vi "Frame_to_word_14444B.vi"() -> ()   [LabVIEW 2019]
uses:
  <vilib>/addons/Modulation/Analog/support/mod_Set Error Source.vi
  <vilib>/addons/Modulation/Digital/Support/Common/Validators/mod_Generate Filter Coefficients Validate.vi
  <vilib>/addons/Modulation/Digital/General/subVIs/mod_Generate Filter Coefficients.vi
  <vilib>/addons/Modulation/Digital/General/MT Generate ASK system parameters (M).vi
  <vilib>/addons/Modulation/Analog/MT Modulate AM (DSB).vi
  <vilib>/addons/Modulation/Analog/MT Upconvert Baseband (Real).vi
  <vilib>/measure/macond.llb/IIR Filter for 1 Chan.vi
  <vilib>/express/express analysis/Spectral/Block/exnSpectralBlock spectral measurements RMS poly.vi
  <vilib>/express/express analysis/Spectral/Block/exnSpectralBlock spectral measurements RMS WFM.vi
  <vilib>/addons/Modulation/Analog/MT Downconvert Passband (Real).vi
  <vilib>/addons/Modulation/Analog/MT Demodulate AM (DSB).vi
  <vilib>/ErrorRing/Error Ring.xnode
  <vilib>/express/express analysis/Spectral/XNode/ExpressSpectralMeasurementsBlockNode.xnode
  <vilib>/addons/Modulation/niAMT.lvlib
  <vilib>/measure/NI_MAPro.lvlib
  <vilib>/addons/Modulation/niDMT.lvlib
panel:
  out "lo(x)":u8 format="%x"
  out "hi(x)":u8 format="%x"
  out "Array of byte":u8[](array[numeric]) format="%x"
  out "decode":cluster{"t0":dbl, "dt":dbl, "Y":dbl[]}(graph)
  out "Command":cluster{"t0":dbl, "dt":dbl, "Y":dbl[]}(graph)
  out "DEMODulate":cluster{"t0":dbl, "dt":dbl, "Y":dbl[]}(graph)
  out "spectrum analog signal 6":waveform(dbl)(graph)
  out "spectrum analog signal 5":cluster{"t0":dbl, "dt":dbl, "Y":dbl[]}(graph)
  out "Analog signal 8":waveform(dbl)(graph)
  out "spectrum analog signal 4":cluster{"t0":dbl, "dt":dbl, "Y":dbl[]}(graph)
  out "antenna":waveform(dbl)(graph)
  out "summ":waveform(dbl)(graph)
  out "antenna":waveform(dbl)(graph)
  out "spectrum analog signal 3":cluster{"t0":dbl, "dt":dbl, "Y":dbl[]}(graph)
  out "spectrum analog signal 2":cluster{"t0":dbl, "dt":dbl, "Y":dbl[]}(graph)
  out "spectrum analog signal":cluster{"t0":dbl, "dt":dbl, "Y":dbl[]}(graph)
  out "Video  without CRC":cluster{"t0":dbl, "dt":dbl, "Y":dbl[]}(graph)
  in  "AFi":u8[](array[numeric])=[2] format="%x"
  in  "APf":u8[](array[numeric])=[5] format="%x"
  out "SOF+DATA+EOF":cluster{"t0":dbl, "dt":dbl, "Y":dbl[]}(graph)
  out "Video":cluster{"t0":dbl, "dt":dbl, "Y":dbl[]}(graph)
  out "video NRZ":cluster{"t0":dbl, "dt":dbl, "Y":dbl[]}(graph)
  in  "command":enum16{"WUPB", "REQB"}(ring)
  in  "CARRIER (hz)":dbl
  in  "BIT RATE":dbl
  out "10% ASK":waveform(dbl)(graph)
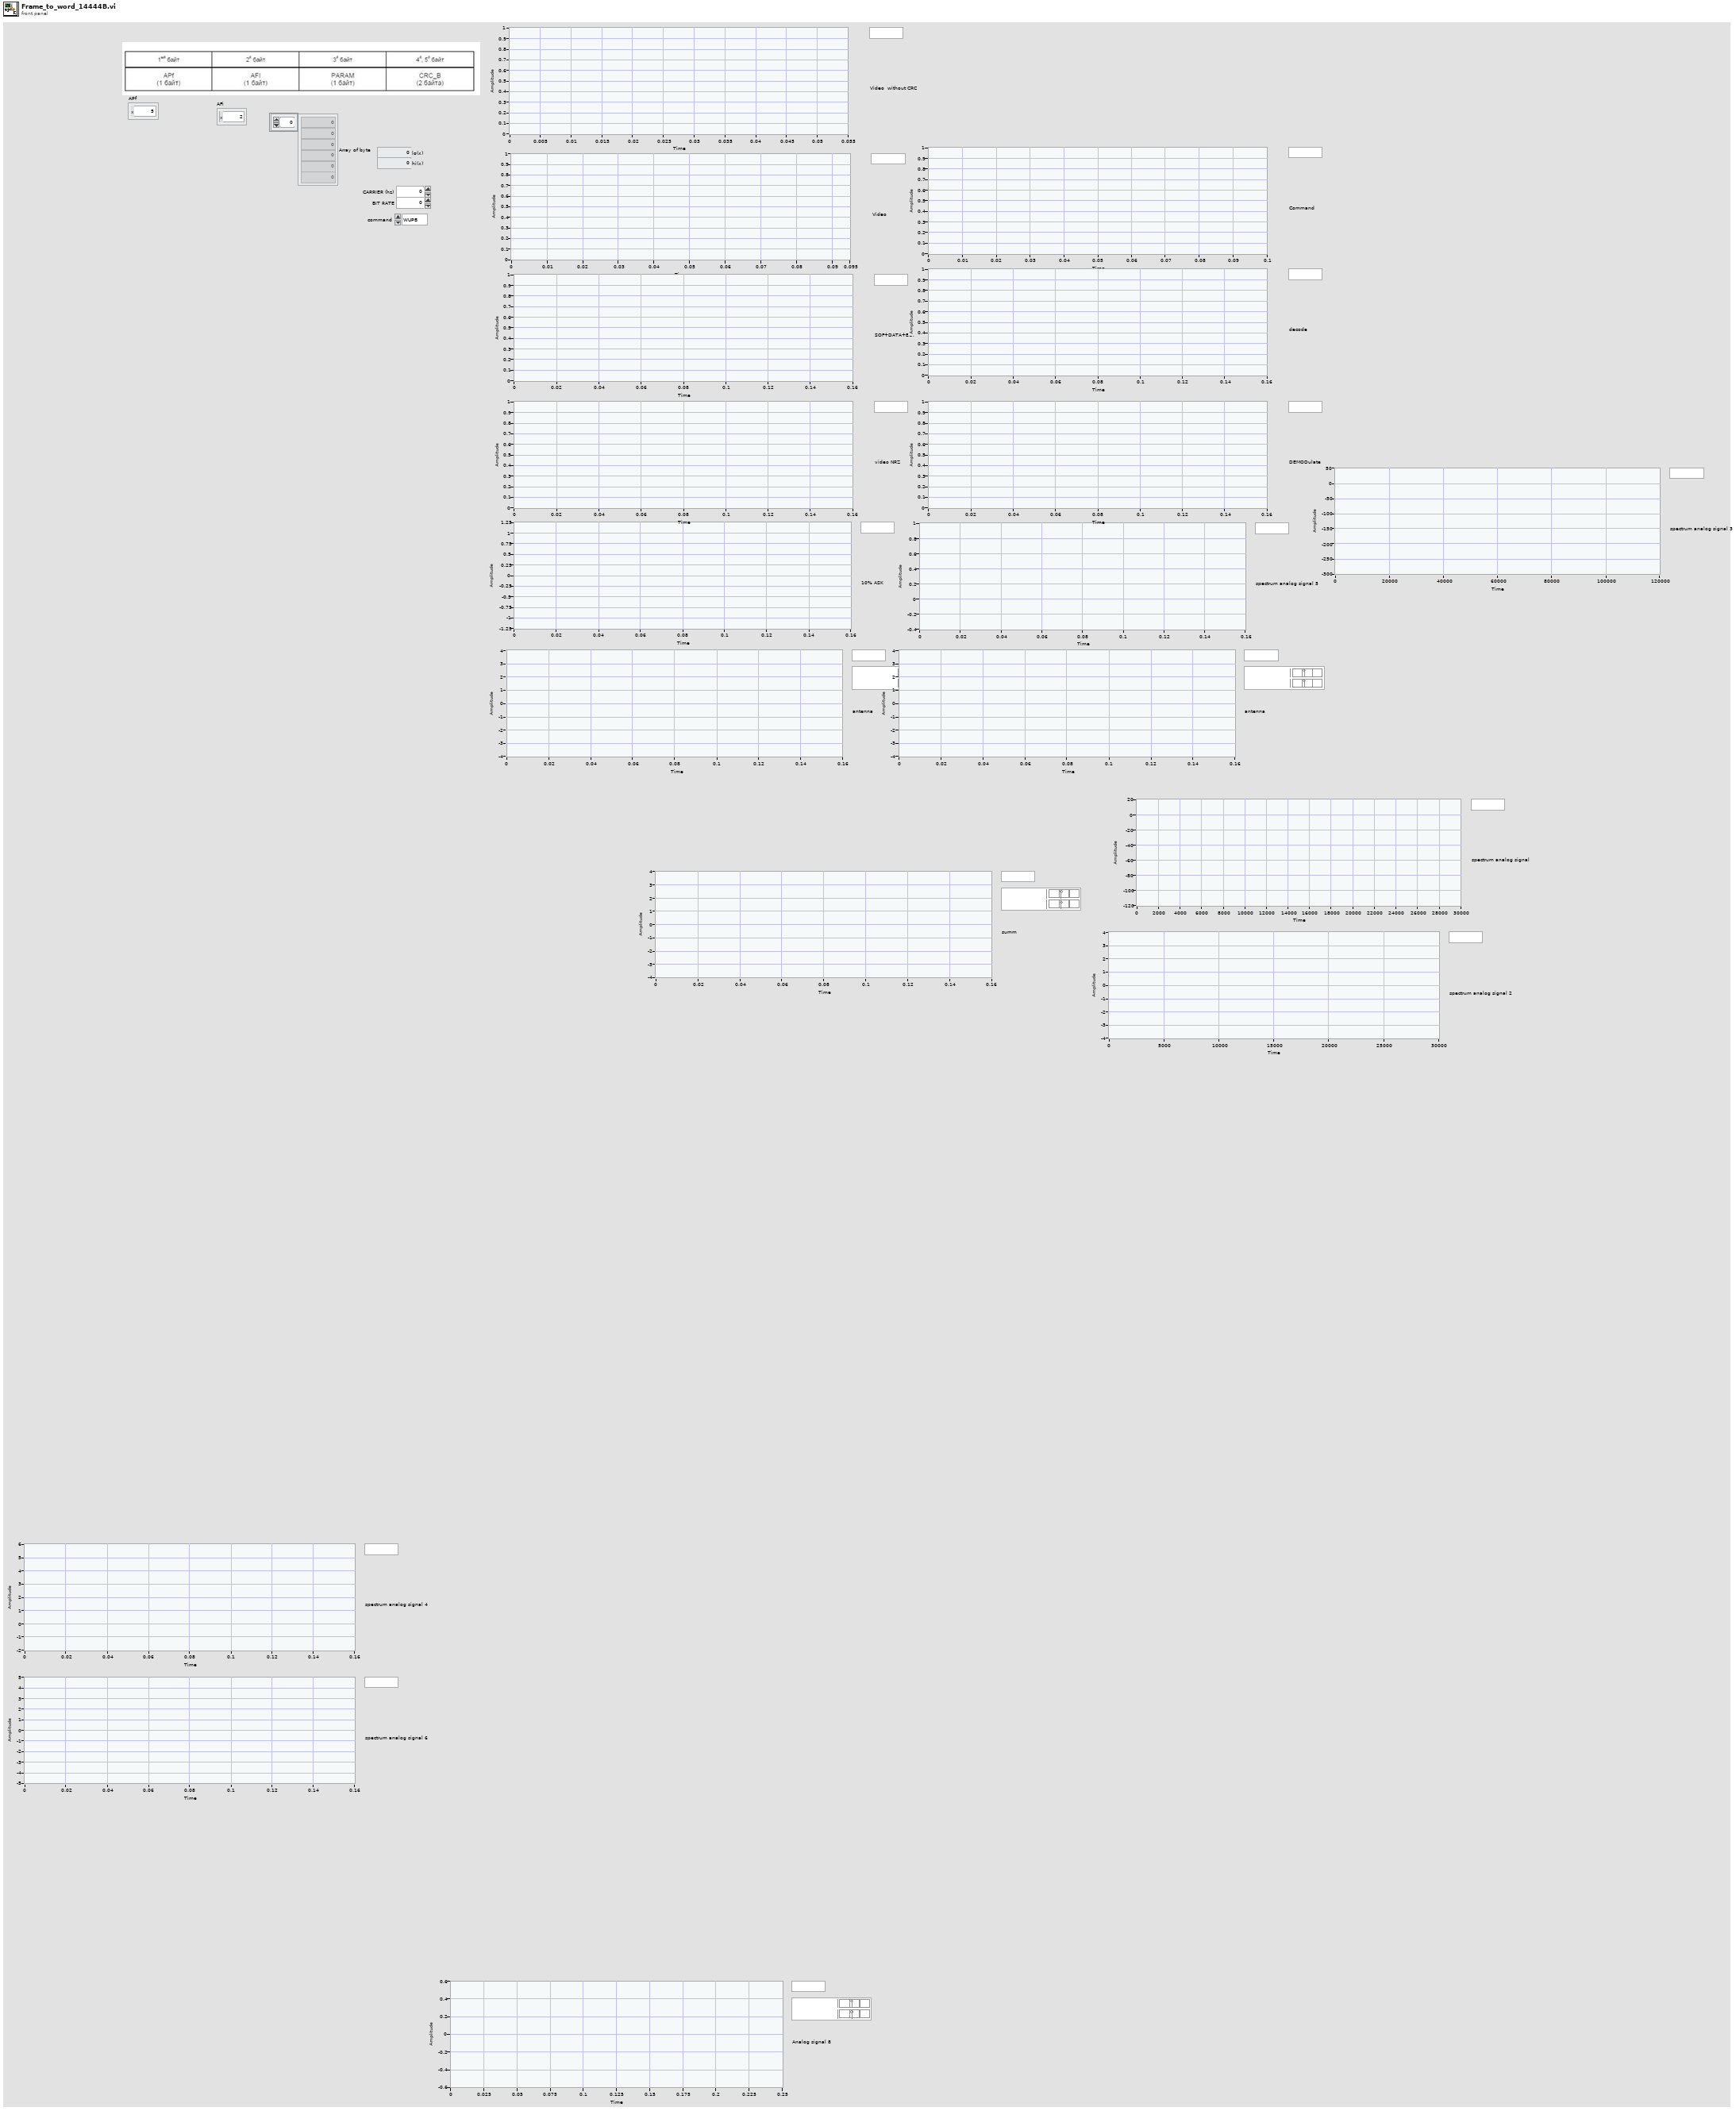
[diagram p1: front panel]
types:
  T1 = enum16{"none", "Raised Cosine", "Root Raised Cos", "Gaussian"}
  T2 = enum16{"FSK", "PSK", "QAM", "MSK", "PAM", "ASK", "CPM"}
  T3 = cluster{"Topology":enum16{"Off", "Butterworth", "Chebyshev", "Inverse Chebyshev", "Elliptic", "Bessel"}, "Type":enum16{"Lowpass", "Highpass", "Bandpass", "Bandstop"}, "Order":i32, "Lower Fc":dbl, "Upper Fc":dbl, "PB Ripple":dbl, "SB Attenuation":dbl}
  T4 = cluster{"passband ripple (dB)":dbl, "stopband start (Hz)":dbl, "stopband gain (dB)":dbl, "compute filter stopband ? (T)":bool}
  T5 = typedef "niAMT.lvlib/Complex Data Waveform.ctl" = cluster{"t0":dbl, "dt":dbl, "Y":cdb[]}
  T6 = cluster{"samples per symbol (16)":i32, "symbol map":cdb[]}
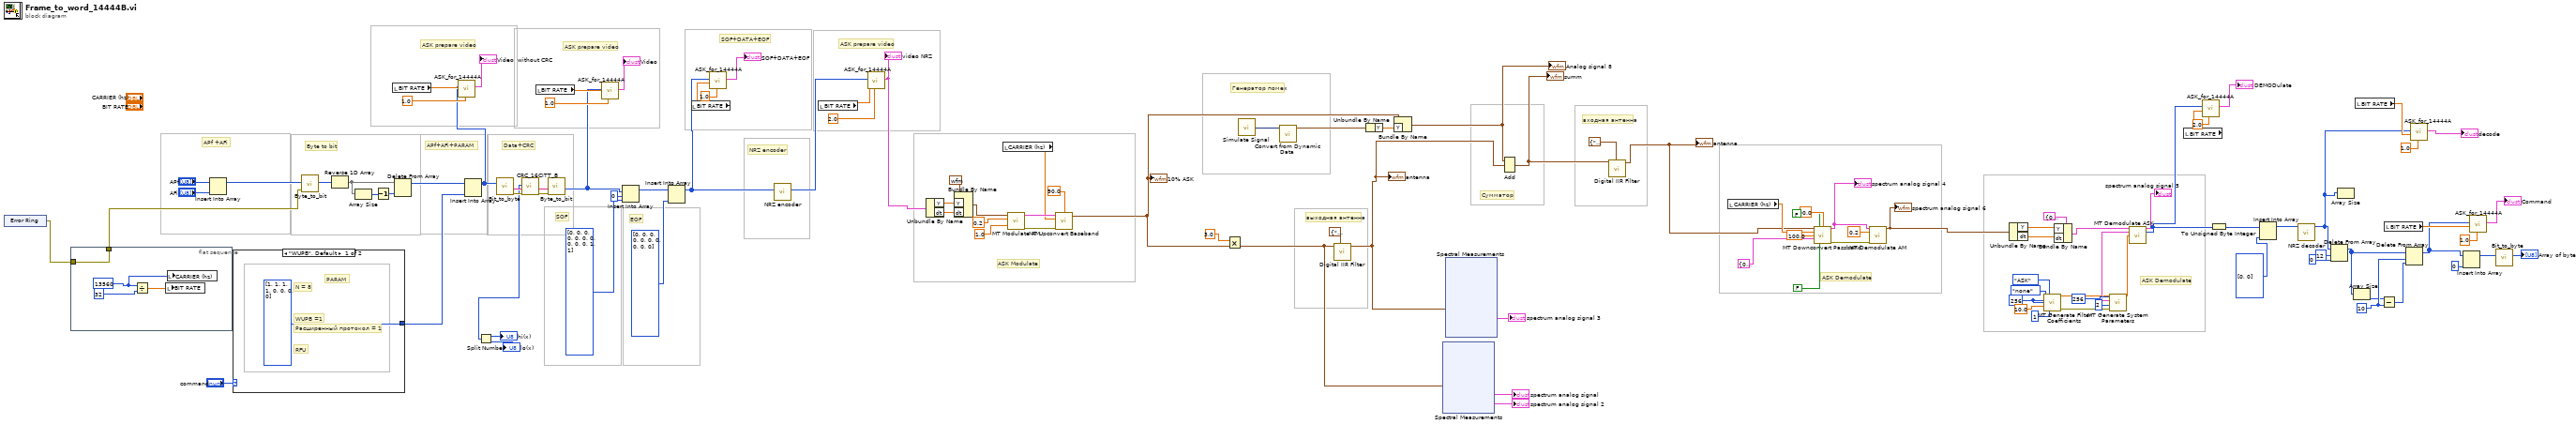
[diagram p0: block diagram]
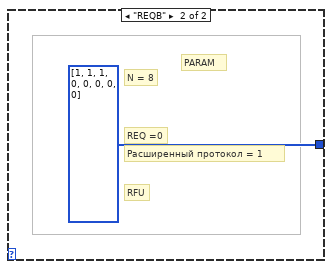
[diagram p2: hidden frame]
diagram:
  w19 = 10 ("length")
  w50 = 256 ("pulse shaping samples per symbol (16)")
  # "ASK Demodulate"
  # "ASK Demodulate"
  # "входная антенна"
  # "Сумматор"
  # "выходная антенна"
  # "Генератор помех"
  # "ASK prepare video"
  # "Data+CRC"
  # "APf+AFi+PARAM"
  # "APf +AFi"
  # "ASK Modulate"
  # "SOF+DATA+EOF"
  # "EOF"
  # "SOF"
  # "ASK prepare video"
  # "ASK prepare video"
  # "NRZ encoder"
  # "Byte to bit"
  n1 = xnode "Error Ring"() -> ("error out"=w88:errorcluster)
  n2 = flat-sequence {
    tunnel: w88 -> [w114]
    tunnel: [w114] -> w87
    frame #0 {
      w115 = u32 13560
      n3 = Divide(x=w115, y=u32 32) -> (x/y=w116:dbl)
      n4 = local write "BIT RATE"(w116) -> ()
      n5 = local write "CARRIER (hz)"(w115) -> ()
    }
  }
  n6 = Insert Into Array(array="APf", new element="AFi") -> (w84:u8[])  [unwired: 1 in]
  n7 = case shown="\"WUPB\", Default" "command" {
    tunnel: [u8[] [1, 1, 1, 1, 0, 0, 0, 0] ("AFi 2") u8[] [1, 1, 1, 0, 0, 0, 0, 0] ("AFi 2")] -> w83
    frame "WUPB", Default {
      # "PARAM"
      # "RFU"
      # "Расширенный протокол = 1"
      # "WUPB =1"
      # "N = 8"
    }
    frame "REQB" {
      # "PARAM"
      # "RFU"
      # "Расширенный протокол = 1"
      # "REQ =0"
      # "N = 8"
    }
  }
  n8 = call "Byte_to_bit.vi"("Error In"=w87, "Array of byte"=w84) -> ("Arrray of bit"=w113:u8[])  [unwired: 5 in, 2 out]
  n9 = Reverse 1D Array(array=w113) -> (reversed array=w110:u8[])
  n10 = Array Size(array=w110) -> (size(s)=w109:i32)
  n11 = Decrement(x=w109) -> (x-1=w108:i32)
  n12 = local read "BIT RATE"() -> (w79:dbl)
  n13 = Delete From Array(array=w110, index=w108) -> (array with subset deleted=w78:u8[])  [unwired: 1 in, 1 out]
  n14 = Insert Into Array(array=w78, new element=w83) -> (w77:u8[])  [unwired: 1 in]
  n15 = call "ASK_for_14444A.vi"("encoder divider"=1.0 ("y"), "BIT RATE"=w79, "Bit stream out (NRZ encode)"=w77) -> ("output complex waveform"=→"Video  without CRC":T5)  [unwired: 7 in, 1 out]
  n16 = call "Bit_to_byte.vi"("Array of bit"=w77) -> ("Error Out"=w74:errorcluster, "BYTE"=w73:string)  [unwired: 8 in, 1 out]
  n17 = call "CRC_16CITT_B.vi"("Error In"=w74, "DATA PACKET"=w73) -> ("Error Out"=w82:errorcluster, "DATA PACKET+CRC"=w72:string, "CRC out"=w3:u16)  [unwired: 5 in]
  n18 = Split Number(x=w3) -> (hi(x)=→"hi(x)":u8, lo(x)=→"lo(x)":u8)
  n19 = local read "BIT RATE"() -> (w101:dbl)
  n20 = call "Byte_to_bit.vi"("Error In"=w82, "BYTE"=w72) -> ("Arrray of bit (str)"=w68:u8[])  [unwired: 5 in, 2 out]
  n21 = call "ASK_for_14444A.vi"("encoder divider"=1.0 ("y"), "BIT RATE"=w101, "Bit stream out (NRZ encode)"=w68) -> ("output complex waveform"=→"Video":T5)  [unwired: 7 in, 1 out]
  n22 = Insert Into Array(array=w68, index=0, new element=u8[] [0, 0, 0, 0, 0, 0, 0, 0, 0, 0, 1, 1] ("Bit stream out (NRZ encode)")) -> (w91:u8[])
  n23 = Insert Into Array(array=w91, new element=u8[] [0, 0, 0, 0, 0, 0, 0, 0, 0, 0] ("Bit stream out (NRZ encode)")) -> (w71:u8[])  [unwired: 1 in]
  n24 = local read "BIT RATE"() -> (w96:dbl)
  n25 = call "ASK_for_14444A.vi"("encoder divider"=1.0 ("y"), "BIT RATE"=w96, "Bit stream out (NRZ encode)"=w71) -> ("output complex waveform"=→"SOF+DATA+EOF":T5)  [unwired: 7 in, 1 out]
  n26 = call "NRZ encoder.vi"("Bit stream in"=w71) -> ("Bit stream out (NRZ encode)"=w70:u8[])  [unwired: 9 in, 1 out]
  n27 = local read "BIT RATE"() -> (w112:dbl)
  n28 = call "ASK_for_14444A.vi"("encoder divider"=2.0 ("y"), "BIT RATE"=w112, "Bit stream out (NRZ encode)"=w70) -> ("output complex waveform"=w69:T5)  [unwired: 7 in, 1 out]
  "video NRZ" <- w69
  n29 = Unbundle By Name(w69) -> ("Y"=w93:cdb[], "dt"=w92:dbl)
  n30 = Bundle By Name(cluster=waveform(cdb) {"t0"=timestamp(0 s since 1904-01-01), "dt"=1.0, "Y"=[]} ("waveform"), "Y"=w93, "dt"=w92) -> (w104:waveform(cdb))
  n31 = local read "CARRIER (hz)"() -> (w102:dbl)
  n32 = call-poly <vilib>:"MT Modulate AM.vi"("message signal"=w104, "modulation index"=0.2, "peak message amplitude"=1.0) -> ("AM modulated waveform"=w103:cluster{"t0":dbl, "dt":dbl, "Y":cdb[]}, "error out"=w106:errorcluster)  [unwired: 11 in]
  n33 = call-poly <vilib>:"MT Upconvert Baseband.vi"("baseband waveform (complex)"=w103, "initial phase (deg)"=90.0, "carrier frequency (Hz)"=w102, "error in (no error)"=w106) -> ("passband waveform"=w8:waveform(dbl))  [unwired: 10 in, 1 out]
  "10% ASK" <- w8
  n34 = Multiply(x=3.0, y=w8) -> (x*y=w5:waveform(dbl))
  n35 = call "Simulate Signal"() -> ("Sine with Gaussian Noise"=w63:dynamicdata)  [unwired: 14 in, 1 out]
  n36 = call "Convert from Dynamic Data"("Dynamic Data Type"=w63) -> ("Waveform"=w62:waveform(dbl))  [unwired: 3 in]
  n37 = call-poly <vilib>:"Digital IIR Filter.vi"("IIR filter specifications"=T3 {"Topology"=enum."Butterworth", "Type"=enum."Bandpass", "Order"=3, "Lower Fc"=2000.0, "Upper Fc"=22000.0, "PB Ripple"=1.0, "SB Attenuation"=60.0}, "signal in"=w5) -> ("signal out"=w55:waveform(dbl))  [unwired: 7 in, 2 out]
  "antenna" <- w55
  n38 = Unbundle By Name(w62) -> ("Y"=w61:dbl[])
  n39 = Bundle By Name(cluster=w8, "Y"=w61) -> (w54:waveform(dbl))
  "Analog signal 8" <- w54
  n40 = xnode "Spectral Measurements"("Signals"=w5) -> ("FFT - (RMS)"=→"spectrum analog signal":cluster{"f0":dbl, "df":dbl, "magnitude":dbl[]}, "Phase"=→"spectrum analog signal 2":cluster{"f0":dbl, "df":dbl, "phase":dbl[]})  [unwired: 1 in, 1 out]
  n41 = xnode "Spectral Measurements"("Signals"=w55) -> ("FFT - (RMS)"=→"spectrum analog signal 3":cluster{"f0":dbl, "df":dbl, "magnitude":dbl[]})  [unwired: 1 in, 2 out]
  n42 = Add(1:w55, 2:w54) -> (0:w59:waveform(dbl))  [unwired: 1 in, 1 out]
  "summ" <- w59
  n43 = call-poly <vilib>:"Digital IIR Filter.vi"("IIR filter specifications"=T3 {"Topology"=enum."Butterworth", "Type"=enum."Bandpass", "Order"=3, "Lower Fc"=2000.0, "Upper Fc"=22000.0, "PB Ripple"=1.0, "SB Attenuation"=60.0}, "signal in"=w59) -> ("signal out"=w37:waveform(dbl))  [unwired: 7 in, 2 out]
  "antenna" <- w37
  n44 = local read "CARRIER (hz)"() -> (w58:dbl)
  n45 = call-poly <vilib>:"MT Downconvert Passband.vi"("Waveform"=w37, "reset? (F)"=FALSE, "initial phase (deg)"=90.0, "carrier frequency (Hz)"=w58, "passband bandwidth (Hz)"=100.0, "advanced filter parameters"=T4 {"passband ripple (dB)"=0.01, "stopband start (Hz)"=0.0, "stopband gain (dB)"=-96.0, "compute filter stopband ? (T)"=TRUE}, "enable filter (T)"=FALSE) -> ("downconverted waveform (complex baseband)"=w32:T5, "error out"=w38:errorcluster)  [unwired: 5 in, 2 out]
  "spectrum analog signal 4" <- w32
  n46 = call-poly <vilib>:"MT Demodulate AM.vi"("AM modulated waveform"=w32, "modulation index"=0.2, "error in (no error)"=w38) -> ("AM demodulated waveform"=w36:waveform(dbl))  [unwired: 10 in, 2 out]
  "spectrum analog signal 6" <- w36
  n47 = Unbundle By Name(w36) -> ("Y"=w34:dbl[], "dt"=w33:dbl)
  n48 = call <vilib>:"MT Generate Filter Coefficients.vi"("pulse shaping filter (none)"=T1."none", "modulation type"=T2."ASK", "pulse shaping samples per symbol (16)"=w50, "matched samples per symbol (16)"=w50, "filter parameter"=10.0, "filter length (symbols)"=1) -> ("pulse shaping filter coefficients"=w44:dbl[], "error out"=w47:errorcluster)  [unwired: 1 in, 7 out]
  n49 = Bundle By Name(cluster=cluster{"t0":dbl, "dt":dbl, "Y":dbl[]} {"t0"=0.0, "dt"=0.0, "Y"=[]} ("AM modulated waveform"), "Y"=w34, "dt"=w33) -> (w31:cluster{"t0":dbl, "dt":dbl, "Y":dbl[]})
  n50 = call-poly <vilib>:"MT Generate System Parameters.vi"("samples per symbol (16)"=256, "M-ASK (2)"=2, "error in (no error)"=w47) -> ("ASK system parameters"=w45:T6)  [unwired: 12 out]
  n51 = call <vilib>:"MT Demodulate ASK.vi"("input complex waveform"=w31, "ASK system parameters"=w45, "matched filter coefficients"=w44) -> ("recovered complex waveform"=→"spectrum analog signal 5":T5, "output bit stream"=w25:i8[])  [unwired: 8 in, 3 out]
  n52 = local read "BIT RATE"() -> (w28:dbl)
  n53 = call "ASK_for_14444A.vi"("encoder divider"=2.0 ("y"), "BIT RATE"=w28, "Bit stream out (NRZ encode)"=w25) -> ("output complex waveform"=→"DEMODulate":T5)  [unwired: 7 in, 1 out]
  n54 = To Unsigned Byte Integer(number=w25) -> (unsigned 8bit integer=w15:u8[])
  n55 = Insert Into Array(array=w15, new element=u8[] [0, 0]) -> (w7:u8[])  [unwired: 1 in]
  n56 = call "NRZ decoder.vi"("Bit stream in"=w7) -> ("Array"=w6:u8[])  [unwired: 9 in, 1 out]
  n57 = Delete From Array(array=w6, length=12, index=0) -> (array with subset deleted=w21:u8[])  [unwired: 1 out]
  n58 = Array Size(array=w6) -> ()  [unwired: 1 out]
  n59 = Array Size(array=w21) -> (size(s)=w17:i32)
  n60 = local read "BIT RATE"() -> (w27:dbl)
  n61 = Subtract(x=w17, y=w19) -> (x-y=w18:i32)
  n62 = local read "BIT RATE"() -> (w22:dbl)
  n63 = Delete From Array(array=w21, length=w19, index=w18) -> (array with subset deleted=w12:u8[])  [unwired: 1 out]
  n64 = call "ASK_for_14444A.vi"("encoder divider"=1.0 ("y"), "BIT RATE"=w27, "Bit stream out (NRZ encode)"=w6) -> ("output complex waveform"=→"decode":T5)  [unwired: 7 in, 1 out]
  n65 = Insert Into Array(array=w12, new element=u8 0 ("new element/subarray")) -> (w10:u8[])  [unwired: 1 in]
  n66 = call "ASK_for_14444A.vi"("encoder divider"=1.0 ("y"), "BIT RATE"=w22, "Bit stream out (NRZ encode)"=w12) -> ("output complex waveform"=→"Command":T5)  [unwired: 7 in, 1 out]
  n67 = call "Bit_to_byte.vi"("Array of bit"=w10) -> ("Array of byte"=→"Array of byte":u8[])  [unwired: 8 in, 2 out]
